vi "System Semaphore Open.vi"(8 "error in (no error)":errorcluster, 11 "Name":string="LabVIEW_System_Semaphore") -> (0 "error out":errorcluster, 3 "Handle":u16 format="%.0x")   [LabVIEW 2011]
uses:
  kernel32.dll
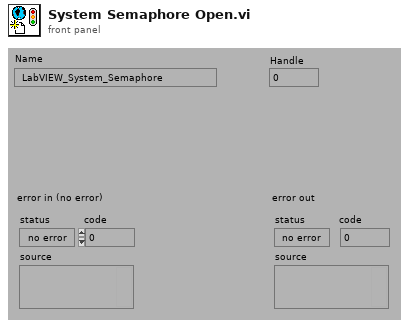
[diagram p1: front panel]
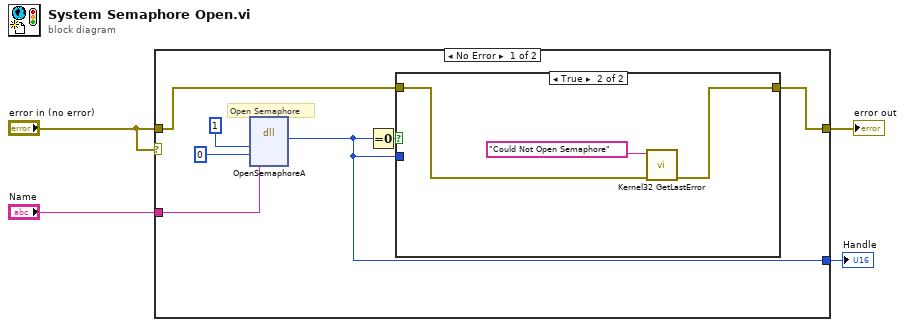
[diagram p0: block diagram]
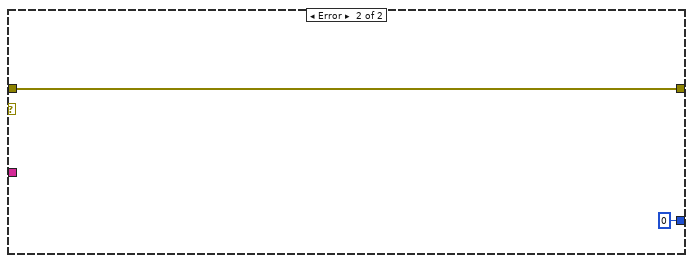
[diagram p3: hidden frame]
diagram:
  n1 = case shown="No Error" "error in (no error)" {
    tunnel: "error in (no error)" -> [w11 w17]
    tunnel: [w10 w17] -> w3
    tunnel: "Name" -> [w6 _]
    tunnel: [w8 0] -> w2
    frame No Error {
      # "Open Semaphore"
      n2 = dll-call lib="kernel32.dll" fn="OpenSemaphoreA"("dwDesiredaccess"=u16 1 ("SecurityDescriptor"), "bininherit"=u32 0 ("SecurityDescriptor"), "name"=w6) -> ("return type"=w8:u16)  [unwired: 6 in, 2 out]
      n3 = Equal To 0?(x=w8) -> (x = 0?=w9:bool)
      n4 = case shown="True" w9 {
        tunnel: w11 -> [w12 w14]
        tunnel: [w12 w13] -> w10
        tunnel: w8 -> [_ _]
        frame False {
          # "No Error"
        }
        frame True {
          n5 = call "Kernel32 GetLastError.vi"("error in (no error)"=w14, "Message"="Could Not Open Semaphore" ("source")) -> ("error out"=w13:errorcluster)  [unwired: 9 out]
        }
      }
    }
    frame Error {
      (unwired) FALSE
    }
  }
  "error out" <- w3
  "Handle" <- w2
